vi "delete bad files.vi"(8 "error in (no error)":errorcluster, 11 "Array":path[](array[path])) -> (0 "error out":errorcluster)   [LabVIEW 2013]
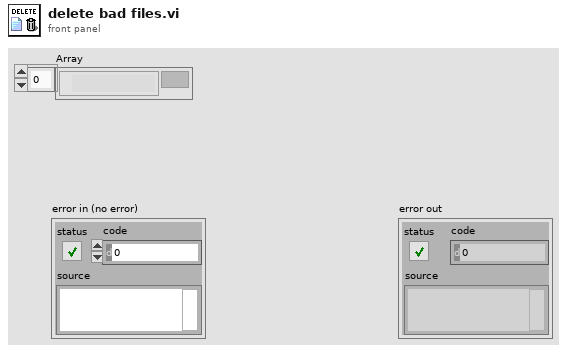
[diagram p1: front panel]
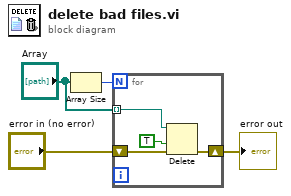
[diagram p0: block diagram]
diagram:
  n1 = Array Size(array="Array") -> (size(s)=w2:i32)
  n2 = for {
    N: w2 -> [_]
    tunnel: "Array" -> [w8] mode=indexing
    shift-right: [w6] -> w4
    shift-left: "error in (no error)" -> [w5]
    n3 = Delete(path (use dialog)=w8, confirm (F)=TRUE, error in=w5) -> (error out=w6:errorcluster)  [unwired: 2 in, 2 out]
  }
  "error out" <- w4
